vi "Dashboard Main.vi"() -> ()   [LabVIEW 2019]
uses:
  <vilib>/Utility/miscctls.llb/LVRowAndColumnTypeDef.ctl
  <vilib>/event_ctls.llb/eventvkey.ctl
  <vilib>/Rock Robotics/Network Tables/NT Read Numeric Array.vi
  <vilib>/Rock Robotics/Network Tables/NT Read Boolean.vi
  <vilib>/Rock Robotics/Network Tables/NT Read Variant.vi
  <vilib>/Rock Robotics/WPI/Dashboard/WPI_DashboardLogging Global.vi
panel:
  in  "Camera Settings Right":T1={"Frame Rate"=30, "Compression"=30, "Size"=1, "DB Camera Config"=FALSE} {"Frame Rate" scale=1.0..30.0; "Compression" scale=100.0..-1.0; "Size" items=["640x480", "320x240", "160x120"]}
  in  "Camera Name Right":string(combo)="No Camera Selection"
  out "Camera Perf":string
  in  "Camera Settings":T1={"Frame Rate"=30, "Compression"=30, "Size"=1, "DB Camera Config"=FALSE} {"Frame Rate" scale=1.0..30.0; "Compression" scale=100.0..-1.0; "Size" items=["640x480", "320x240", "160x120"]}
  in  "TCP":refnum<k5>
  in  "Rec Mode":enum32{"Stop", "Record", "Playback"}(radio)
  out "Robot IP":string
  out "Image Message":string="Timeout in Camera Communications"
  in  "Dashboard Tab":T2(tab)
  in  "Select Auto":string(combo)="Select Autonomous ..."
  out "NT Connection":bool
  out "MotorChart R":cluster{"Numeric":dbl, "Numeric":dbl}(graph)
  out "MotorChart L":cluster{"Numeric":dbl, "Numeric":dbl}(graph)
  out "MotorSliders R":cluster{"MotorSlide1":dbl, "MotorSlide2":dbl} {"MotorSlide2" scale=-1.0..1.0 scale format="%#_2e"; "MotorSlide1" scale=-1.0..1.0 scale format="%#_2e"}
  out "MotorSliders L":cluster{"MotorSlide1":dbl, "MotorSlide2":dbl} {"MotorSlide2" scale=-1.0..1.0 scale format="%#_2e"; "MotorSlide1" scale=-1.0..1.0 scale format="%#_2e"}
  out "Gyro":dbl(knob) scale=0.0..360.0
  out "JS1 Z":dbl(slide) scale=-1.0..1.0 scale format="%#_2e"
  out "JS1 Graph":cluster{"X":dbl, "Y":dbl}[](graph)
  out "JS1 Buttons":T3
  out "JS2 Z":dbl(slide) scale=-1.0..1.0 scale format="%#_2e"
  out "JS2 Graph":cluster{"X":dbl, "Y":dbl}[](graph)
  out "JS2 Buttons":T3
  out "Mode":T4(ring)=enum."Auto Disabled"
  out "Right Camera Perf":cluster{"Bandwidth (Mbps)":dbl, "FPS":dbl}
  out "Camera Image Right":T5(plugin-control)
  in  "DB/String 9":string
  in  "DB/String 8":string
  in  "DB/String 7":string
  in  "DB/String 6":string
  in  "DB/String 5":string
  in  "DB/String 4":string
  in  "DB/String 3":string
  in  "DB/String 2":string
  in  "DB/String 1":string
  in  "DB/String 0":string
  in  "DB/Slider 0":dbl(slide) scale=0.0..5.0
  in  "DB/Slider 1":dbl(slide) scale=0.0..5.0
  in  "DB/Slider 2":dbl(slide) scale=0.0..5.0
  in  "DB/Slider 3":dbl(slide) scale=0.0..5.0
  out "DB/LED 3":bool
  out "DB/LED 2":bool
  out "DB/LED 1":bool
  out "DB/LED 0":bool
  in  "DB/Button 3":bool
  in  "DB/Button 2":bool
  in  "DB/Button 1":bool
  in  "DB/Button 0":bool caption="New Name"
  out "Unjam?":bool
  out "Turret State":T6
  out "Safe for Trench?":bool
  out "Feeder State":T7
  in  "Test Slider":dbl(slide) scale=0.0..100.0 scale format="%#_3g"
  in  "On/Off":bool caption="Solenoid"
  in  "Test Name":u16(ring) items=["Select the test to run..."]
  in  "Test Tree":string(tree)
  in  "Motor":cluster{"Value":dbl, "Enable":bool} {"Value" scale=-1.0..1.0 scale format="%#_3g"}
  out "Progress":T8 {"Test Progress" scale=0.0..100.0}
  in  "Rev/Fwd":cluster{"Forward":bool, "Reverse":bool}
  in  "Test Ring":u16(ring) items=["Monochrome", "Color"]
  out "Cmd Status":string
  in  "Execute Command":bool
  in  "Command Params":string[][](table)
  in  "Command Selection":i32(listbox)
  in  "CheckList":i32(listbox)
  out "Tree":string(tree)
  out "Camera Image":T5(plugin-control)
  out "Background":bool
  in  "Camera Name":string(combo)="No Camera Selection"
  # "HW"
  # "HW"
  # "Joysticks"
  # "Drive Motors"
  # "Front"
  # "Right"
  # "Left"
  # "Back"
  # "Safe for Trench?"
  # "Feeder State"
  # "Turret State"
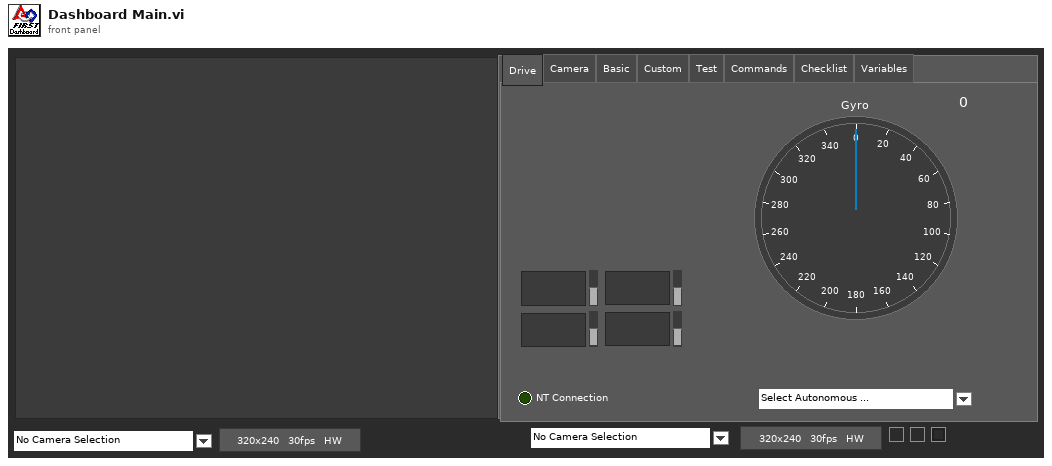
[diagram p1: front panel]
types:
  T1 = cluster{"Frame Rate":i32, "Compression":i32, "Size":u16, "DB Camera Config":bool}
  T2 = enum32{"Drive", "Camera", "Basic", "Custom", "Test", "Commands", "Checklist", "Variables"}
  T3 = cluster{bool, bool, bool, bool, bool, bool, bool, bool, bool, bool, bool, bool}
  T4 = enum8{"Tele-Op Disabled", "Tele-Op Enabled", "Auto Disabled", "Auto Enabled", "Test Disabled", "Test Enabled", "Disconnected", "No Code", "E-Stop"}
  T5 = typedef "IMAQ Image.ctl" = refnum<image>
  T6 = cluster{"Shooter Up To Speed?":bool, "Aligned With Target?":bool, "Hood at Angle?":bool, "Shooting?":bool, "Hood Angle":dbl, "Turret Angle":dbl, "Shooter Velocity":dbl}
  T7 = cluster{"Feeder Up to Speed? ":bool, "Index Clear?":bool}
  T8 = cluster{"Test Progress":u8, "Test Progress Text":string}
  T9 = cluster{"Save Path":path, "Interval (s)":dbl, "Keep":i32}
  T10 = typedef "Image Type" = u32
  T11 = cluster{"IDs":cluster{"RPC field ID":u16, "Unique ID":u16}, "String":string}
  T12 = cluster{"Error Strings":string, "Disable Counts":cluster{u16, u16}, "Rail Faults":cluster{u16, u16, u16}, "Robot IP":string, "DB Mode":u8, "Event Info":cluster{"Name":string, "Type":u8, "Number":u16, "Replay":u8}}
  T13 = cluster{"Storage":cluster{"Disk Free":u64, "RAM Block":u32, "RAM free":u32}, "CPU Utilization":cluster{"CPU % ISR":sgl, "CPU % Time Crit":sgl, "CPU % Timed Str":sgl, "CPU % High":sgl, "CPU % Above":sgl, "CPU % Normal":sgl, "CPU % Low":sgl}, "CAN":cluster{"% Bus Utilization":sgl, "Bus Off Cnt":u32, "TX_FIFO Full Cnt":u32, "Receive Error Cnt":u8, "Transmit Error Cnt":u8}, "HID":cluster{"HID Outputs":u32, "Rumble Low":u16, "Rumble High":u16}[]}
  T14 = cluster{"Status bits":cluster{"Test Mode":bool, "Autonomous":bool, "Enabled":bool, "Code Start":bool, "Brownout":bool, "Reserved 2":bool, "Reserved 3":bool, "E-Stop":bool}, "Code Trace":cluster{"Disabled":bool, "TeleOp":bool, "Auto":bool, "Test":bool}, "Controller Type":enum16{"unknown", "cRIO", "roboRio"}, "Code?":enum16{"unknown", "noCode", "code"}, "Battery V":dbl}
  T15 = cluster{"Control Bits":cluster{"TestMode":bool, "Autonomous":bool, "Enabled":bool, "FMS Present":bool, bool, bool, bool, "E-Stop":bool}, "Team Station ":u8, "Countdown":sgl, "Joystick Values":cluster{"Axes":dbl[], "Buttons":bool[], "POVs":i16[]}[]}
  T16 = cluster{"Axes":dbl[], "Buttons":bool[], "POVs":i16[]}[]
  T17 = cluster{"Axes":dbl[], "Buttons":bool[], "POVs":i16[]}
  T18 = cluster{"Buttons[0]":bool, "Buttons[1]":bool, "Buttons[2]":bool, "Buttons[3]":bool, "Buttons[4]":bool, "Buttons[5]":bool, "Buttons[6]":bool, "Buttons[7]":bool, "Buttons[8]":bool, "Buttons[9]":bool, "Buttons[10]":bool, "Buttons[11]":bool}
  T19 = cluster{"Camera Image":refnum<vi>, "Dashboard Tab":refnum<vi>, "Background":refnum<vi>, "Rec Mode":refnum<vi>, "Test Slider":refnum<vi>, "On/Off ":refnum<vi>, "Test Ring":refnum<vi>, "Rev/Fwd":refnum<vi>, "Test Name":refnum<vi>, "Motor":refnum<vi>, "Progress":refnum<vi>, "CheckList":refnum<vi>, "Tree":refnum<vi>, "Test Tree":refnum<vi>, "Command Params":refnum<vi>, "Command Selection":refnum<vi>, "Execute Command":refnum<vi>, "Cmd Status":refnum<vi>, "Camera Settings":refnum<vi>, "Camera Name":refnum<vi>, "Camera Perf":refnum<vi>, "Camera Settings Right":refnum<vi>, "Camera Name Right":refnum<vi>, "Camera Image Right":refnum<vi>}
  T20 = cluster{"Global Rectangle":i32[], "Contours":cluster{"Contour Type":u32, "ROI Type":u32, "Points":i32[]}[]}
  T21 = cluster{"Camera Name":string, string, "Saved DB Images Info":cluster{"Save Path":path, "Interval (s)":dbl, "Keep":i32}}
  T22 = cluster{"Camera Name Right":string, string, "Saved DB Images Info":cluster{"Save Path":path, "Interval (s)":dbl, "Keep":i32}}
  T23 = cluster{"Operation":enum16{"Update", "Clear"}, "Color Box":u32}[]
  T24 = typedef "eventvkey.ctl" = enum16{"ASCII", "Enter", "Return", "Shift", "Ctrl", "Alt", "Cmd", "Opt", "Caps", "NumLock", "Clear", "Break", "Up", "Down", "Left", "Right", "Insert", "Delete", "Home", "End", "PageUp", "PageDown", "Escape", "Help", "Pause", "ScrollLock", "F1", "F2", "F3", "F4", "F5", "F6", "F7", "F8", "F9", "F10", "F11", "F12", "F13", "F14", "F15", "F16", "F17", "F18", "F19", "F20", "F21", "F22", "F23", "F24", "Play", "VolumeUp", "VolumeDown", "Mute", "Two Byte Char"}
  T25 = cluster{"Image Size":bool, "Image Type":bool, "Pixel Value":bool, "ROI Information":bool, "Zoom Factor":bool}
  T26 = cluster{"Operation":enum16{"Update", "Clear"}, "Color Box":u32}
  T27 = typedef "LVRowAndColumnTypeDef.ctl" = cluster{"Row":i32, "Column":i32}
  T28 = cluster{"Shift":bool, "Ctrl":bool, "Alt":bool, "Cmd":bool, "Opt":bool}
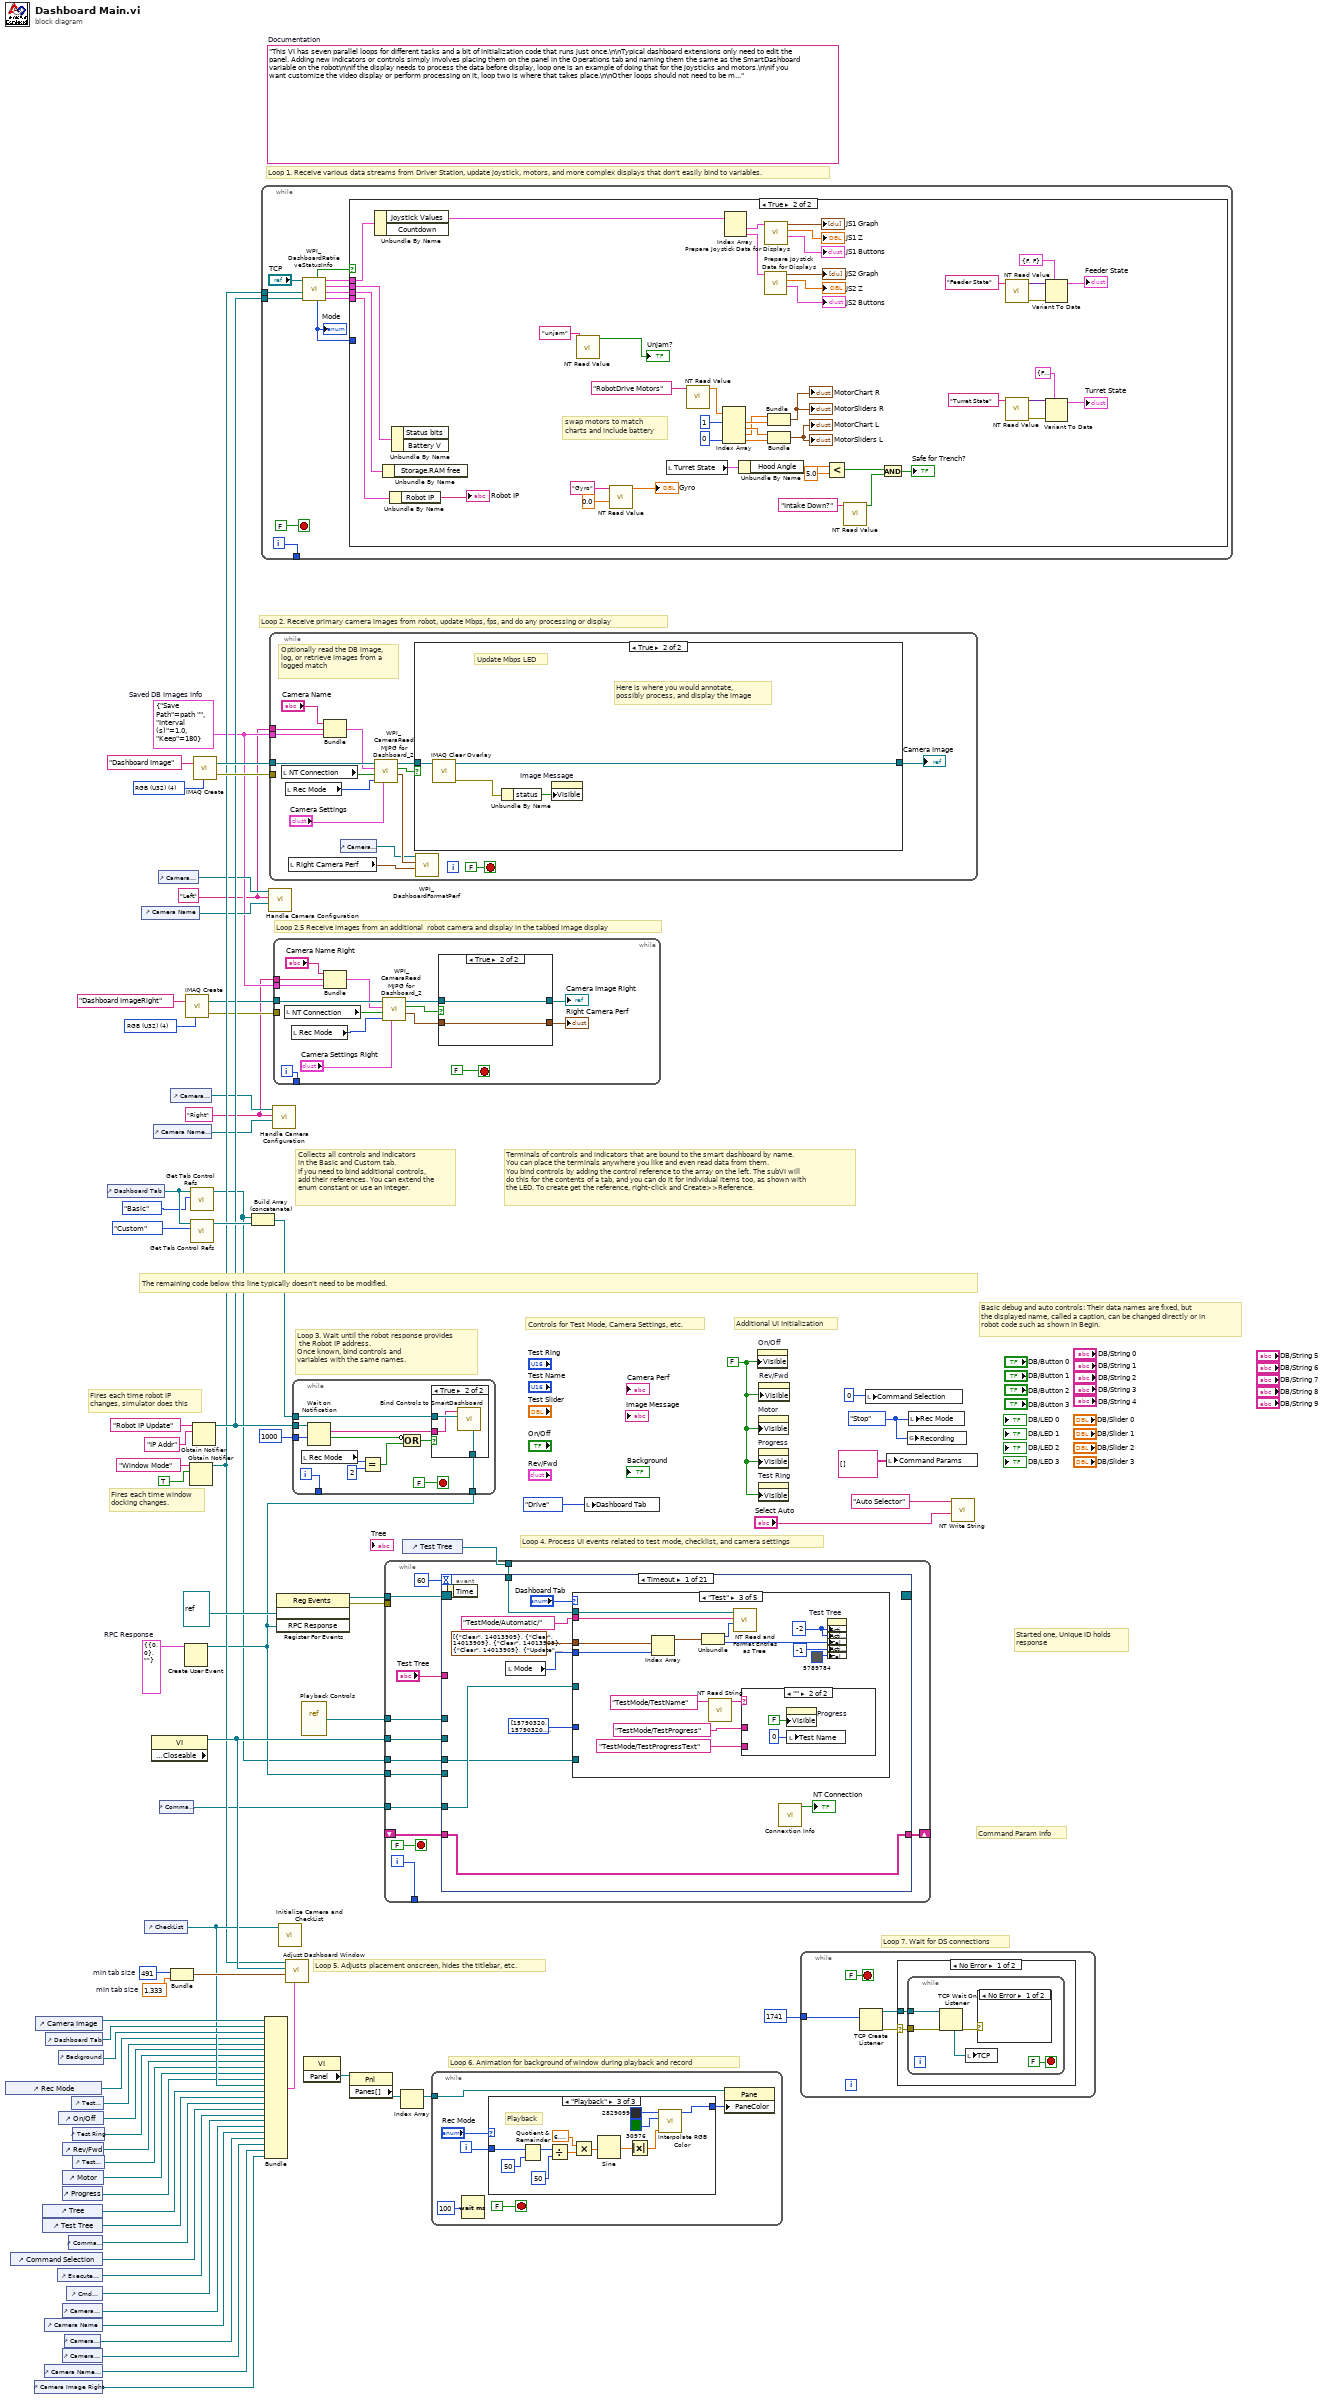
[diagram p0: block diagram]
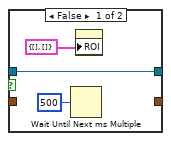
[diagram p2: hidden frame]
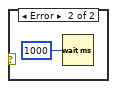
[diagram p3: hidden frame]
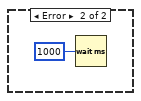
[diagram p4: hidden frame]
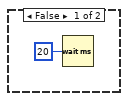
[diagram p5: hidden frame]
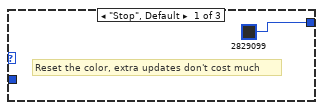
[diagram p6: hidden frame]
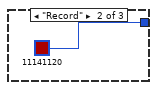
[diagram p7: hidden frame]
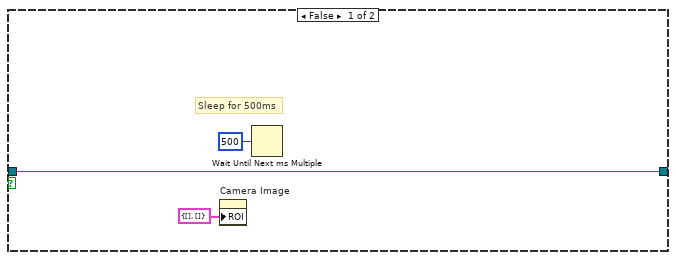
[diagram p9: hidden frame]
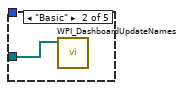
[diagram p11: hidden frame]
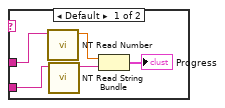
[diagram p12: hidden frame]
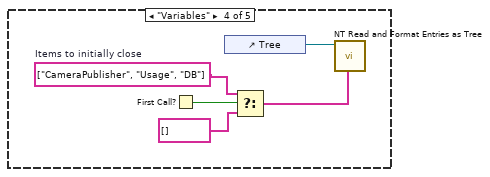
[diagram p13: hidden frame]
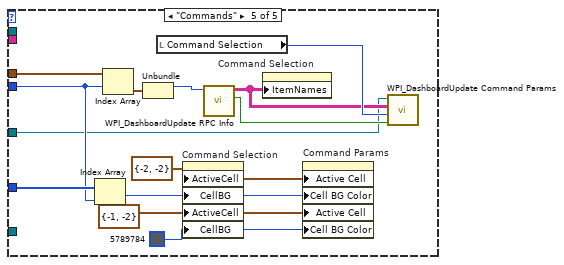
[diagram p14: hidden frame]
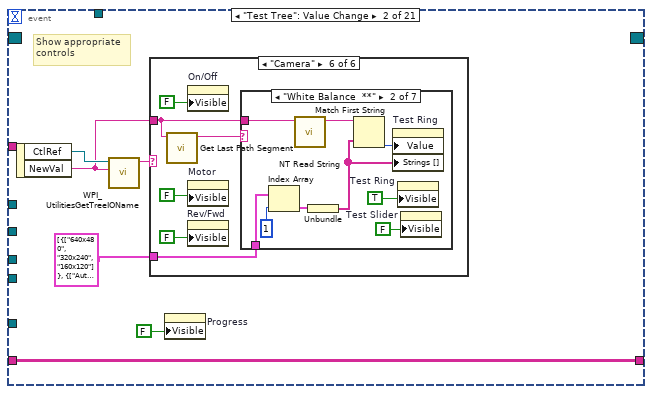
[diagram p15: hidden frame]
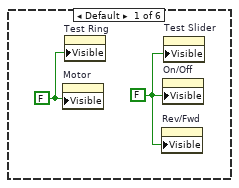
[diagram p16: hidden frame]
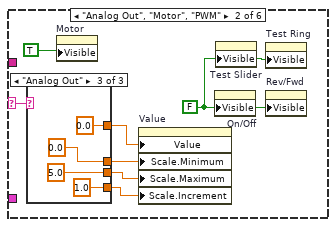
[diagram p17: hidden frame]
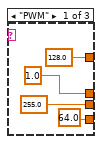
[diagram p18: hidden frame]
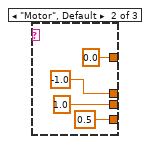
[diagram p19: hidden frame]
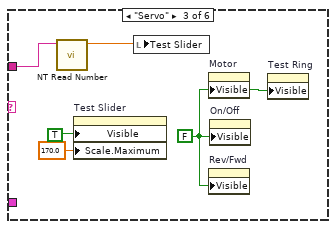
[diagram p20: hidden frame]
diagram:
  w3 = T9 {"Save Path"=path "", "Interval (s)"=1.0, "Keep"=180}  # Saved DB Images Info
  w2 = "Right"
  w1 = "Left"
  w13 = T10 4 items=["Grayscale (U8)", "Grayscale (I16)", "Grayscale (SGL)", "Complex (CSG)", "RGB (U32)", "HSL (U32)", "RGB (U64)"] ("Image Type")
  w29 = T11 {"IDs"={"RPC field ID"=0, "Unique ID"=0}, "String"=""}  # RPC Response
  w52 = 491  # min tab size
  w51 = 1.333  # min tab size
  w59 = enum32{"Stop", "Record", "Playback"}."Stop" ("Rec Mode")
  w36 = FALSE ("Visible")
  (unwired) "This VI has seven parallel loops for different tasks and a bit of initialization code that runs just once.\n\nTypical dashboard extensions only need to edit the panel. Adding new indicators or controls simply involves placing them on the panel in the Operations tab and naming them the same as the SmartDashboard variable on the robot\n\nIf the display needs to process the data before display, loop one is an example of doing that for the joysticks and motors.\n\nIf you want customize the video display or perform processing on it, loop two is where that takes place.\n\nOther loops should not need to be modified. They are pretty standard, and document the task they perform."  # Documentation
  w76 = T10 4 items=["Grayscale (U8)", "Grayscale (I16)", "Grayscale (SGL)", "Complex (CSG)", "RGB (U32)", "HSL (U32)", "RGB (U64)"] ("Image Type")
  # "Loop 2.5 Receive images from an additional  robot camera and display in the tabbed image display"
  # "Command Param Info"
  # "Started one, Unique ID holds\nresponse"
  # "Loop 7. Wait for DS connections"
  # "Basic debug and auto controls: Their data names are fixed, but\nthe displayed name, called a caption, can be changed directly or in\nrobot code such as shown in Begin."
  # "Controls for Test Mode, Camera Settings, etc."
  # "Additional UI Initialization"
  # "Loop 6. Animation for background of window during playback and record"
  # "Fires each time robot IP\nchanges, simulator does this"
  # "Fires each time window\ndocking changes."
  # "Collects all controls and indicators\nin the Basic and Custom tab.\nIf you need to bind additional controls,\nadd their references. You can extend the\nenum constant or use an integer."
  # "The remaining code below this line typically doesn't need to be modified."
  # "Loop 4. Process UI events related to test mode, checklist, and camera settings"
  # "Terminals of controls and indicators that are bound to the smart dashboard by name.\nYou can place the terminals anywhere you like and even read data from them.\nYou bind controls by adding the control reference to the array on the left. The subVI will\ndo this for the contents of a tab, and you can do it for individual items too, as shown with\nthe LED. To create get the reference, right-click and Create>>Reference."
  # "Loop 3. Wait until the robot response provides\n the Robot IP address.\nOnce known, bind controls and\nvariables with the same names."
  # "Loop 5. Adjusts placement onscreen, hides the titlebar, etc."
  # "Loop 1. Receive various data streams from Driver Station, update joystick, motors, and more complex displays that don't easily bind to variables."
  # "Loop 2. Receive primary camera images from robot, update Mbps, fps, and do any processing or display"
  n1 = control-ref of="Rec Mode"() -> (w42:refnum<vi>)
  n2 = control-ref of="Command Selection"() -> (w28:refnum<vi>)
  n3 = control-ref of="Camera Image Right"() -> (w6:refnum<vi>)
  n4 = control-ref of="Camera Image"() -> (w54:refnum<vi>)
  n5 = control-ref of="Tree"() -> (w46:refnum<vi>)
  n6 = control-ref of="Test Tree"() -> (w45:refnum<vi>)
  n7 = control-ref of="Camera Name"() -> (w19:refnum<vi>)
  n8 = control-ref of="Camera Name Right"() -> (w7:refnum<vi>)
  n9 = control-ref of="Dashboard Tab"() -> (w53:refnum<vi>)
  n10 = control-ref of="Execute Command"() -> (w30:refnum<vi>)
  n11 = control-ref of="Background"() -> (w49:refnum<vi>)
  n12 = control-ref of="On/Off"() -> (w40:refnum<vi>)
  n13 = control-ref of="Progress"() -> (w37:refnum<vi>)
  n14 = control-ref of="Camera Settings"() -> (w20:refnum<vi>)
  n15 = control-ref of="Camera Settings Right"() -> (w8:refnum<vi>)
  n16 = control-ref of="Rev/Fwd"() -> (w38:refnum<vi>)
  n17 = control-ref of="Motor"() -> (w43:refnum<vi>)
  n18 = control-ref of="Camera Perf"() -> (w18:refnum<vi>)
  n19 = control-ref of="Cmd Status"() -> (w24:refnum<vi>)
  n20 = control-ref of="Command Params"() -> (w31:refnum<vi>)
  n21 = control-ref of="Test Slider"() -> (w41:refnum<vi>)
  n22 = control-ref of="Test Ring"() -> (w39:refnum<vi>)
  n23 = control-ref of="Test Name"() -> (w44:refnum<vi>)
  n24 = control-ref of="Dashboard Tab"() -> (w57:refnum<vi>)
  n25 = control-ref of="Camera Name"() -> (w21:refnum<vi>)
  n26 = control-ref of="CheckList"() -> (w47:refnum<vi>)
  n27 = property class="VI" props=["Front Panel.Closeable"]() -> (reference out=w58:refnum<vi>)  [unwired: 2 in, 2 out]
  n28 = control-ref of="Camera Name Right"() -> (w9:refnum<vi>)
  n29 = control-ref of="Camera Settings"() -> (w22:refnum<vi>)
  n30 = control-ref of="Command Params"() -> (w23:refnum<vi>)
  n31 = control-ref of="Camera Settings Right"() -> (w10:refnum<vi>)
  n32 = Bundle("min tab size"=w52, "min tab size"=w51) -> (w50:cluster{"min tab size":i32, "min tab size":dbl})  [unwired: 1 in]
  n33 = Create User Event(user event datatype=w29) -> (user event=w25:refnum<user-event>)  [unwired: 1 in, 1 out]
  n34 = call "IMAQ Create"("Image Name"="Dashboard ImageRight", "Image Type"=w13) -> ("New Image"=w12:T5, "error out"=w11:errorcluster)  [unwired: 2 in, 1 out]
  n35 = Obtain Notifier(name (unnamed)="Window Mode", notification data type=TRUE) -> (notifier out=w34:refnum<notifier>)  [unwired: 2 in, 2 out]
  n36 = call <vilib>:"Get Tab Control Refs.vi"("Page Index"=T2."Basic" ("Dashboard Tab"), "TabControl in"=w57) -> ("ControlsOnPage"=w17:refnum<vi>[])  [unwired: 9 in]
  n37 = call <vilib>:"Get Tab Control Refs.vi"("Page Index"=T2."Custom" ("Dashboard Tab"), "TabControl in"=w57) -> ("ControlsOnPage"=w56:refnum<vi>[])  [unwired: 9 in]
  n38 = Obtain Notifier(name (unnamed)="Robot IP Update", notification data type="IP Addr" ("name (unnamed)")) -> (notifier out=w35:refnum<notifier>)  [unwired: 2 in, 2 out]
  n39 = call "IMAQ Create"("Image Name"="Dashboard Image", "Image Type"=w76) -> ("New Image"=w74:T5, "error out"=w73:errorcluster)  [unwired: 2 in, 1 out]
  n40 = Build Array (concatenate)(w17, w56) -> (w55:refnum<vi>[])
  n41 = while {
    tunnel: [w86] -> _
    tunnel: w35 -> [w80]
    tunnel: w34 -> [w77]
    i -> [w86]
    stop <- FALSE stop-if-true
    n42 = call <vilib>:"WPI_DashboardRetrieveStatusInfo.vi"("Binding Refnum"=w80, "Window Mode Notifier"=w77, "TCP Cnx"="TCP") -> ("Power and Errors"=w81:T12, "Robot Metrics"=w84:T13, "Status Info"=w85:T14, "Control Info"=w82:T15, "Robot Mode"=w79:T4, "Process?"=w83:bool)  [unwired: 3 in]
    "Mode" <- w79
    n43 = case shown="True" w83 {
      tunnel: w85 -> [_ w134]
      tunnel: w84 -> [_ w133]
      tunnel: w82 -> [_ w132]
      tunnel: w81 -> [_ w131]
      tunnel: w79 -> [_ _]
      frame False {
        n44 = Wait (ms)(milliseconds to wait=u32 20) -> ()  [unwired: 1 out]
      }
      frame True {
        # "swap motors to match\ncharts and include battery"
        n45 = Unbundle By Name(w132) -> ("Joystick Values"=w122:T16)  [unwired: 1 out]
        n46 = Unbundle By Name(w133) -> ()  [unwired: 1 out]
        n47 = Unbundle By Name(w131) -> ("Robot IP"=→"Robot IP":string)
        n48 = Unbundle By Name(w134) -> ()  [unwired: 2 out]
        n49 = call-poly <vilib>:"NT Read Value.vi"("Name"="unjam") -> ("Boolean"=→"Unjam?":bool)  [unwired: 9 in, 1 out]
        n50 = call-poly <vilib>:"NT Read Value.vi"("Default Value"=0.0, "Name"="Gyro") -> ("Numeric"=→"Gyro":dbl)  [unwired: 8 in, 1 out]
        n51 = local read "Turret State"() -> (w95:T6)
        n52 = call-poly <vilib>:"NT Read Value.vi"("Name"="RobotDrive Motors") -> ("Numeric Array"=w112:dbl[])  [unwired: 9 in, 1 out]
        n53 = Index Array(array=w112, index #1=1, index #4=0) -> (element #1=w126:dbl, element #2=w127:dbl, element #3=w125:dbl, element #4=w130:dbl)  [unwired: 2 in]
        n54 = Index Array(array=w122) -> (element #1=w121:T17, element #2=w117:T17)  [unwired: 2 in]
        n55 = Unbundle By Name(w95) -> ("Hood Angle"=w93:dbl)
        n56 = call "Prepare Joystick Data for Displays.vi"("Joystick Values"=w117) -> ("Buttons"=→"JS2 Buttons":T18, "Z Axis"=→"JS2 Z":dbl, "Cartesian Data"=→"JS2 Graph":cluster{"X axis":dbl, "X axis":dbl}[])  [unwired: 8 in]
        n57 = call "Prepare Joystick Data for Displays.vi"("Joystick Values"=w121) -> ("Buttons"=→"JS1 Buttons":T18, "Z Axis"=→"JS1 Z":dbl, "Cartesian Data"=→"JS1 Graph":cluster{"X axis":dbl, "X axis":dbl}[])  [unwired: 8 in]
        n58 = Bundle("Numeric"=w125, "Numeric"=w126) -> (→"MotorChart R" →"MotorSliders R":cluster{"Numeric":dbl, "Numeric":dbl})  [unwired: 1 in]
        n59 = Bundle("Numeric"=w127, "Numeric"=w130) -> (→"MotorChart L" →"MotorSliders L":cluster{"Numeric":dbl, "Numeric":dbl})  [unwired: 1 in]
        n60 = Less?(x=w93, y=5.0) -> (x < y?=w91:bool)
        n61 = call-poly <vilib>:"NT Read Value.vi"("Name"="Intake Down?") -> ("Boolean"=w106:bool)  [unwired: 9 in, 1 out]
        n62 = And(x=w91, y=w106) -> (x .and. y?=→"Safe for Trench?":bool)
        n63 = call-poly <vilib>:"NT Read Value.vi"("Name"="Feeder State") -> ("error out"=w98:errorcluster, "Variant"=w104:variant)  [unwired: 9 in]
        n64 = call-poly <vilib>:"NT Read Value.vi"("Name"="Turret State") -> ("error out"=w99:errorcluster, "Variant"=w100:variant)  [unwired: 9 in]
        n65 = Variant To Data(error in=w98, type=T7 {"Feeder Up to Speed? "=FALSE, "Index Clear?"=FALSE} ("Feeder State"), Variant=w104) -> (data=→"Feeder State":T7)  [unwired: 1 out]
        n66 = Variant To Data(error in=w99, type=T6 {"Shooter Up To Speed?"=FALSE, "Aligned With Target?"=FALSE, "Hood at Angle?"=FALSE, "Shooting?"=FALSE, "Hood Angle"=0.0, "Turret Angle"=0.0, "Shooter Velocity"=0.0} ("Turret State"), Variant=w100) -> (data=→"Turret State":T6)  [unwired: 1 out]
      }
    }
  }
  n67 = Bundle("Camera Image"=w54, "Dashboard Tab"=w53, "Background"=w49, "Rec Mode"=w42, "Test Slider"=w41, "On/Off"=w40, "Test Ring"=w39, "Rev/Fwd"=w38, "Test Name"=w44, "Motor"=w43, "Progress"=w37, "CheckList"=w47, "Tree"=w46, "Test Tree"=w45, "Command Params"=w31, "Command Selection"=w28, "Execute Command"=w30, "Cmd Status"=w24, "Camera Settings"=w20, "Camera Name"=w19, "Camera Perf"=w18, "Camera Settings Right"=w8, "Camera Name Right"=w7, "Camera Image Right"=w6) -> (w48:T19)  [unwired: 1 in]
  n68 = call "Handle Camera Configuration.vi"("CameraNameRef"=w21, "Display Name"=w1, "ClusterRef"=w22) -> ()  [unwired: 9 in]
  n69 = while {
    tunnel: w74 -> [w148]
    tunnel: w73 -> [_]
    tunnel: w3 -> [w141]
    tunnel: w1 -> [w138]
    stop <- FALSE stop-if-true
    # "Optionally read the DB image,\nlog, or retrieve images from a\nlogged match"
    n70 = local read "NT Connection"() -> (w142:bool)
    n71 = local read "Rec Mode"() -> (w145:enum32{"Stop", "Record", "Playback"})
    n72 = local read "Right Camera Perf"() -> (w136:cluster{"Bandwidth (Mbps)":dbl, "FPS":dbl})
    n73 = Bundle("Camera Name"="Camera Name", w138, "Saved DB Images Info"=w141) -> (w140:T21)  [unwired: 1 in]
    n74 = control-ref of="Camera Perf"() -> (w135:refnum<vi>)
    n75 = call <vilib>:"WPI_CameraRead MJPG for Dashboard_2.vi"("Camera Settings"="Camera Settings", "Rec Mode"=w145, "NT Connection"=w142, "Capture Info"=w140, "Image in"=w148) -> ("perf info"=w137:cluster{"Bandwidth (Mbps)":dbl, "fps":dbl}, "Active"=w146:bool, "Image\\ out"=w147:T5)  [unwired: 4 in]
    n76 = case shown="True" w146 {
      tunnel: w147 -> [w151 w154]
      tunnel: [w151 w153] -> w143
      frame False {
        # "Sleep for 500ms"
        n77 = property on="Camera Image" class="ImageControl"("ROI"=T20 {"Global Rectangle"=[], "Contours"=[]}) -> ()  [unwired: 2 in, 2 out]
        n78 = Wait Until Next ms Multiple(millisecond multiple=u32 500) -> ()  [unwired: 1 out]
      }
      frame True {
        # "Here is where you would annotate,\npossibly process, and display the image"
        # "Update Mbps LED"
        n79 = call "IMAQ Clear Overlay"("Image"=w154) -> ("error out"=w155:errorcluster, "Image Out"=w153:T5)  [unwired: 2 in, 7 out]
        n80 = Unbundle By Name(w155) -> ("status"=w156:bool)
        n81 = property on="Image Message" class="Str"("Visible"=w156) -> ()  [unwired: 2 in, 2 out]
      }
    }
    "Camera Image" <- w143
    n82 = call <vilib>:"WPI_DashboardFormatPerf.vi"("Right Camera Perf"=w136, "Performance"=w137, "String in"=w135) -> ()  [unwired: 9 in]
  }
  n83 = call "Handle Camera Configuration.vi"("CameraNameRef"=w9, "Display Name"=w2, "ClusterRef"=w10) -> ()  [unwired: 9 in]
  n84 = while {
    tunnel: w12 -> [w171]
    tunnel: w11 -> [_]
    tunnel: [w166] -> _
    tunnel: w3 -> [w162]
    tunnel: w2 -> [w159]
    i -> [w166]
    stop <- FALSE stop-if-true
    n85 = local read "NT Connection"() -> (w163:bool)
    n86 = local read "Rec Mode"() -> (w170:enum32{"Stop", "Record", "Playback"})
    n87 = Bundle("Camera Name Right"="Camera Name Right", w159, "Saved DB Images Info"=w162) -> (w161:T22)  [unwired: 1 in]
    n88 = call <vilib>:"WPI_CameraRead MJPG for Dashboard_2.vi"("Camera Settings"="Camera Settings Right", "Rec Mode"=w170, "NT Connection"=w163, "Capture Info"=w161, "Image in"=w171) -> ("perf info"=w157:cluster{"Bandwidth (Mbps)":dbl, "fps":dbl}, "Active"=w165:bool, "Image\\ out"=w168:T5)  [unwired: 4 in]
    n89 = case shown="True" w165 {
      tunnel: w168 -> [w173 w176]
      tunnel: [w173 w176] -> w164
      tunnel: [_ w175] -> w158
      tunnel: w157 -> [_ w175]
      frame False {
        n90 = Wait Until Next ms Multiple(millisecond multiple=u32 500) -> ()  [unwired: 1 out]
        n91 = property on="Camera Image Right" class="ImageControl"("ROI"=T20 {"Global Rectangle"=[], "Contours"=[]}) -> ()  [unwired: 2 in, 2 out]
      }
      frame True {
      }
    }
    "Camera Image Right" <- w164
    "Right Camera Perf" <- w158
  }
  n92 = register-events(refnum<vi> refnum, w25) -> (reference out=w63:refnum<event-registration>, error out=w62:errorcluster)  [unwired: 2 in]
  n93 = call "Initialize Camera and CheckList.vi"("ListBox in"=w47) -> ()  [unwired: 11 in]
  n94 = call "Adjust Dashboard Window.vi"("Sizing Refnums"=w48, "Size Constraints"=w50, "VI"=w58, "WIn Mode"=w34) -> ()  [unwired: 8 in]
  n95 = while {
    tunnel: w55 -> [w188]
    tunnel: w35 -> [w186]
    tunnel: [w184] -> _
    tunnel: u32 1000 ("milliseconds to wait") -> [w183]
    tunnel: w25 -> [w177]
    i -> [w184]
    stop <- FALSE stop-if-true
    n96 = local read "Rec Mode"() -> (w179:enum32{"Stop", "Record", "Playback"})
    n97 = Wait on Notification(notifier=w186, timeout in ms (-1)=w183) -> (notification=w185:string, timed out?=w181:bool)  [unwired: 2 in, 2 out]
    n98 = Equal?(x=w179, y=u16 2 ("Rec Mode")) -> (x = y?=w180:bool)
    n99 = Compound Arithmetic op=OR(invert w181, w180) -> (w182:bool)
    n100 = case shown="True" w182 {
      tunnel: w188 -> [_ w191]
      tunnel: w185 -> [_ w190]
      tunnel: w177 -> [_ w189]
      frame False {
      }
      frame True {
        n101 = call <vilib>:"Bind Controls to SmartDashboard.vi"("RPC ref"=w189, "Bound Control Refs"=w191, "Server IP Address"=w190) -> ()  [unwired: 9 in]
      }
    }
  }
  n102 = vi-ref "Playback Controls.vi"() -> (w64:refnum<vi>)
  n103 = property class="VI"() -> ("Panel"=w66:refnum<vi>)  [unwired: 2 in, 2 out]
  n104 = property class="Pnl"(reference=w66) -> ("Panes[]"=w67:refnum<vi>[])  [unwired: 1 in, 2 out]
  n105 = Index Array(array=w67) -> (element=w65:refnum<vi>)  [unwired: 1 in]
  n106 = control-ref of="Test Tree"() -> (w68:refnum<vi>)
  n107 = while {
    tunnel: [w201] -> _
    tunnel: w68 -> [w200]
    tunnel: w64 -> [w199]
    tunnel: w63 -> [w198]
    tunnel: w62 -> [_]
    tunnel: w58 -> [w197]
    tunnel: w25 -> [w196]
    tunnel: w23 -> [w195]
    shift-right: [w194] -> _
    shift-left: _ -> [w193]
    tunnel: w17 -> [w192]
    i -> [w201]
    stop <- FALSE stop-if-true
    n108 = event shown="[0] Timeout" {
      selector: w198 -> [_ _ _ _ _ _ _ _ _ _ _ _ _ _ _ _ _ _ _ _ _]
      dyn-events: [_ _ _ _ _ _ _ _ _ _ _ _ _ _ _ _ w461 _ _ _ _] -> _
      timeout: u32 60 ("milliseconds to wait") -> [_ _ _ _ _ _ _ _ _ _ _ _ _ _ _ _ _ _ _ _ _]
      tunnel: w200 -> [w213 _ _ _ _ _ _ _ _ _ _ _ _ _ _ _ _ _ _ _ _]
      tunnel: "Test Tree" -> [_ _ _ _ _ _ _ _ _ _ _ w428 w436 w438 w442 w450 _ _ _ _ _]
      tunnel: w199 -> [_ _ _ _ _ _ _ _ _ _ _ _ _ _ _ _ w463 _ w481 _ _]
      tunnel: w197 -> [_ _ _ _ _ _ _ _ _ _ _ _ _ _ _ _ w459 _ _ _ _]
      tunnel: w196 -> [_ _ _ _ _ _ _ _ _ _ _ _ _ _ _ _ w457 _ _ _ _]
      tunnel: w195 -> [w208 _ _ _ _ _ w379 _ _ _ _ _ _ _ _ _ _ _ _ _ _]
      tunnel: [w207 w256 w358 w363 w372 w376 w377 w386 w396 w403 w415 w427 w434 w437 w441 w449 w456 w476 w478 w482 w495] -> w194
      tunnel: w193 -> [w207 w256 w358 w363 w372 w376 w377 _ _ w403 w415 w427 w434 w437 w441 w449 w456 w476 w478 w482 w495]
      tunnel: w192 -> [w205 _ _ _ _ _ _ _ _ _ _ _ _ _ _ _ _ _ _ _ _]
      event Timeout {
        n109 = event-data() -> ()  [unwired: 1 in, 1 out]
        n110 = local read "Mode"() -> (w210:T4)
        n111 = case shown="\"Test\"" "Dashboard Tab" {
          tunnel: w213 -> [_ _ w229 _ _]
          tunnel: "TestMode/Automatic/" ("Name Pattern") -> [_ _ w228 _ _]
          tunnel: T23 [{"Operation"=enum."Clear", "Color Box"=14013909}, {"Operation"=enum."Clear", "Color Box"=14013909}, {"Operation"=enum."Clear", "Color Box"=14013909}, {"Operation"=enum."Clear", "Color Box"=14013909}, {"Operation"=enum."Update", "Color Box"=14013909}, {"Operation"=enum."Update", "Color Box"=16777215}, {"Operation"=enum."Clear", "Color Box"=14013909}, {"Operation"=enum."Clear", "Color Box"=14013909}, {"Operation"=enum."Clear", "Color Box"=14013909}] -> [_ _ w221 _ w249]
          tunnel: w210 -> [_ _ w220 _ w248]
          tunnel: u32[] [15790320, 15790320, 15790320, 15790320, 16777215, 16777215, 15790320, 15790320, 15790320] -> [_ _ _ _ w254]
          tunnel: w208 -> [_ _ _ _ w242]
          tunnel: w205 -> [_ w215 _ _ _]
          frame "Custom", Default {
          }
          frame "Basic" {
            n112 = call <vilib>:"WPI_DashboardUpdateNames.vi"("Controls on Tab"=w215) -> ()  [unwired: 11 in]
          }
          frame "Test" {
            w227 = -2 ("Active Item:Row Number")
            n113 = Index Array(array=w221, index=w220) -> (element=w222:T26)
            n114 = Unbundle(w222) -> ("Operation"=w223:enum16{"Update", "Clear"}, "Color Box"=w224:u32)
            n115 = call <vilib>:"NT Read String.vi"("Name"="TestMode/TestName") -> ("String"=w218:string)  [unwired: 9 in, 1 out]
            n116 = call <vilib>:"NT Read and Format Entries as Tree.vi"("Operation"=w223, "Name Pattern"=w228, "Tree Refnum"=w229) -> ()  [unwired: 7 in, 2 out]
            n117 = case shown="\"\"" w218 {
              tunnel: "TestMode/TestProgress" ("Name") -> [w231 _]
              tunnel: "TestMode/TestProgressText" ("Name") -> [w230 _]
              frame Default {
                n118 = call <vilib>:"NT Read Number.vi"("Name"=w231) -> ("Numeric"=w232:dbl)  [unwired: 9 in, 1 out]
                n119 = call <vilib>:"NT Read String.vi"("Name"=w230) -> ("String"=w233:string)  [unwired: 9 in, 1 out]
                n120 = Bundle("Numeric"=w232, "String"=w233) -> (→"Progress":cluster{"Numeric":dbl, "String":string})  [unwired: 1 in]
              }
              frame "" {
                n121 = property on="Progress" class="Clust (strict)"("Visible"=FALSE) -> ()  [unwired: 2 in, 2 out]
                n122 = local write "Test Name"(u16 0) -> ()
              }
            }
            n123 = property on="Test Tree" class="Tree (strict)"("Active Item Row Number"=w227, "ActiveColNum"=w227, "CellBG"=w224, "Active Item Row Number"=-1 ("Active Item:Row Number"), "CellBG"=u32 5789784 ("Color Box")) -> ()  [unwired: 2 in, 2 out]
          }
          frame "Variables" {
            w239 = string[] ["CameraPublisher", "Usage", "DB"]  # Items to initially close
            n124 = First Call?() -> (First Call?: T/F=w240:bool)
            n125 = control-ref of="Tree"() -> (w241:refnum<vi>)
            n126 = Select(t=w239, s=w240, f=string[] []) -> (s? t:f=w237:string[])
            n127 = call <vilib>:"NT Read and Format Entries as Tree.vi"("Tags to  Close"=w237, "Tree Refnum"=w241) -> ()  [unwired: 8 in, 2 out]
          }
          frame "Commands" {
            w250 = u32 5789784 ("Color Box")
            w251 = T27 {"Row"=-1, "Column"=-2} ("Active Cell:Active Cell")
            w253 = T27 {"Row"=-2, "Column"=-2} ("Active Cell:Active Cell")
            n128 = Index Array(array=w254, index=w248) -> (element=w252:u32)
            n129 = Index Array(array=w249, index=w248) -> (element=w247:T26)
            n130 = Unbundle(w247) -> ("Operation"=w246:enum16{"Update", "Clear"})  [unwired: 1 out]
            n131 = local read "Command Selection"() -> (w245:i32)
            n132 = property on="Command Selection" class="MCListbox (strict)"("ActiveCell"=w253, "CellBG"=w252, "ActiveCell"=w251, "CellBG"=w250) -> ()  [unwired: 2 in, 2 out]
            n133 = call <vilib>:"WPI_DashboardUpdate RPC Info.vi"("Operation"=w246) -> ("update"=w244:bool, "commands"=w243:string[][])  [unwired: 9 in]
            n134 = property on="Command Selection" class="MCListbox (strict)"("ItemNames"=w243) -> ()  [unwired: 2 in, 2 out]
            n135 = property on="Command Params" class="Tbl (strict)"("Active Cell"=w253, "Cell BG Color"=w252, "Active Cell"=w251, "Cell BG Color"=w250) -> ()  [unwired: 2 in, 2 out]
            n136 = call <vilib>:"WPI_DashboardUpdate Command Params.vi"("Update"=w244, "NewVal"=w245, "Commands"=w243, "Param Tbl"=w242) -> ()  [unwired: 7 in, 1 out]
          }
        }
        n137 = call <vilib>:"Connextion Info.vi"() -> ("Connected"=→"NT Connection":bool)  [unwired: 10 in, 1 out]
      }
      event "Test Tree": Value Change {
        # "Show appropriate\ncontrols"
        n138 = event-data() -> ("CtlRef"=w259:refnum<vi>, "NewVal"=w257:string)  [unwired: 1 in]
        n139 = call <vilib>:"WPI_UtilitiesGetTreeIOName.vi"("NewVal"=w257, "TreeControl in"=w259) -> ("I/O Name"=w260:string)  [unwired: 9 in]
        n140 = case shown="\"Camera\"" w260 {
          selector: w260 -> [_ w267 _ w289 w298 _]
          tunnel: w257 -> [_ _ w286 w288 _ w305]
          tunnel: cluster{string[]}[] [{["640x480", "320x240", "160x120"]}, {["Auto", "Fixed indoor", "Fixed outdoor 1", "Fixed outdoor 2", "Fixed fluorescent 1", "Fixed fluorescent 2", "Hold current"]}, {["Auto", "Flicker-free 50 Hz", "Flicker-free 60 Hz", "Hold current"]}, {["None", "Prioritize frame rate", "Prioritize image quality"]}, {["Monochrome", "Color"]}] -> [_ _ _ _ _ w304]
          frame Default {
            w262 = FALSE ("Visible")
            w261 = FALSE ("Visible")
            n141 = property on="Motor" class="Clust (strict)"("Visible"=w261) -> ()  [unwired: 2 in, 2 out]
            n142 = property on="Test Ring" class="Ring (strict)"("Visible"=w261) -> ()  [unwired: 2 in, 2 out]
            n143 = property on="Rev/Fwd" class="Clust (strict)"("Visible"=w262) -> ()  [unwired: 2 in, 2 out]
            n144 = property on="On/Off" class="Bool (strict)"("Visible"=w262) -> ()  [unwired: 2 in, 2 out]
            n145 = property on="Test Slider" class="Slide (strict)"("Visible"=w262) -> ()  [unwired: 2 in, 2 out]
          }
          frame "Analog Out", "Motor", "PWM" {
            w268 = FALSE ("Visible")
            n146 = case shown="\"Analog Out\"" w267 {
              tunnel: [1.0 ("Value") -1.0 ("Value") 0.0 ("Value")] -> w266
              tunnel: [255.0 ("Value") 1.0 ("Value") 5.0 ("Value")] -> w265
              tunnel: [128.0 ("Value") 0.0 ("Value") 0.0 ("Value")] -> w264
              tunnel: [64.0 ("Value") 0.5 ("Value") 1.0 ("Value")] -> w263
              frame "PWM" {
              }
              frame "Motor", Default {
              }
              frame "Analog Out" {
              }
            }
            n147 = property on="Motor" class="Clust (strict)"("Visible"=TRUE) -> ()  [unwired: 2 in, 2 out]
            n148 = property on="Value" class="Slide (strict)"("Value"=w264, "Scale.Minimum"=w266, "Scale.Maximum"=w265, "Scale.Increment"=w263) -> ()  [unwired: 2 in, 2 out]
            n149 = property on="On/Off" class="Bool (strict)"("Visible"=w268) -> ()  [unwired: 2 in, 2 out]
            n150 = property on="Test Slider" class="Slide (strict)"("Visible"=w268) -> ()  [unwired: 2 in, 2 out]
            n151 = property on="Test Ring" class="Ring (strict)"("Visible"=w268) -> ()  [unwired: 2 in, 2 out]
            n152 = property on="Rev/Fwd" class="Clust (strict)"("Visible"=w268) -> ()  [unwired: 2 in, 2 out]
          }
          frame "Servo" {
            w284 = FALSE ("Visible")
            n153 = call <vilib>:"NT Read Number.vi"("Name"=w286) -> ("Numeric"=w285:dbl)  [unwired: 9 in, 1 out]
            n154 = property on="Test Slider" class="Slide (strict)"("Visible"=TRUE, "Scale.Maximum"=170.0 ("Scale.Range:Maximum")) -> ()  [unwired: 2 in, 2 out]
            n155 = local write "Test Slider"(w285) -> ()
            n156 = property on="Motor" class="Clust (strict)"("Visible"=w284) -> ()  [unwired: 2 in, 2 out]
            n157 = property on="Rev/Fwd" class="Clust (strict)"("Visible"=w284) -> ()  [unwired: 2 in, 2 out]
            n158 = property on="On/Off" class="Bool (strict)"("Visible"=w284) -> ()  [unwired: 2 in, 2 out]
            n159 = property on="Test Ring" class="Ring (strict)"("Visible"=w284) -> ()  [unwired: 2 in, 2 out]
          }
          frame "Relay", "Solenoid" {
            w287 = FALSE ("Visible")
            n160 = property on="Motor" class="Clust (strict)"("Visible"=w287) -> ()  [unwired: 2 in, 2 out]
            n161 = property on="Test Slider" class="Slide (strict)"("Visible"=w287) -> ()  [unwired: 2 in, 2 out]
            n162 = Search and Replace String(input string=w288, search string="/Value  **", replace string="/Direction") -> (result string=w294:string)  [unwired: 5 in, 3 out]
            n163 = property on="Test Ring" class="Ring (strict)"("Visible"=w287) -> ()  [unwired: 2 in, 2 out]
            n164 = call <vilib>:"NT Read String.vi"("Name"=w294) -> ("String"=w292:string)  [unwired: 9 in, 1 out]
            n165 = Equal?(x="Both directions", y=w292) -> (x = y?=w290:bool)
            n166 = Not(x=w290) -> (.not. x?=w291:bool)
            n167 = property on="Rev/Fwd" class="Clust (strict)"("Visible"=w290) -> ()  [unwired: 2 in, 2 out]
            n168 = property on="On/Off" class="Bool (strict)"("Visible"=w291, "Caption.Text"=w289) -> ()  [unwired: 2 in, 2 out]
          }
          frame "Compressor", "Digital Out" {
            w297 = FALSE ("Visible")
            # "Get direction and finish"
            n169 = property on="Motor" class="Clust (strict)"("Visible"=w297) -> ()  [unwired: 2 in, 2 out]
            n170 = property on="Test Slider" class="Slide (strict)"("Visible"=w297) -> ()  [unwired: 2 in, 2 out]
            n171 = property on="Test Ring" class="Ring (strict)"("Visible"=w297) -> ()  [unwired: 2 in, 2 out]
            n172 = property on="On/Off" class="Bool (strict)"("Visible"=TRUE, "Caption.Text"=w298) -> ()  [unwired: 2 in, 2 out]
            n173 = property on="Rev/Fwd" class="Clust (strict)"("Visible"=FALSE) -> ()  [unwired: 2 in, 2 out]
          }
          frame "Camera" {
            n174 = call <vilib>:"Get Last Path Segment.vi"("String in"=w305) -> ("String out"=w306:string)  [unwired: 10 in]
            n175 = property on="On/Off" class="Bool (strict)"("Visible"=FALSE) -> ()  [unwired: 2 in, 2 out]
            n176 = property on="Motor" class="Clust (strict)"("Visible"=FALSE) -> ()  [unwired: 2 in, 2 out]
            n177 = property on="Rev/Fwd" class="Clust (strict)"("Visible"=FALSE) -> ()  [unwired: 2 in, 2 out]
            n178 = case shown="\"White Balance  **\"" w306 {
              tunnel: w305 -> [w312 w321 w330 w339 w348 _ w354]
              tunnel: w304 -> [w310 w318 w327 w336 w345 _ _]
              frame "Size  **" {
                n179 = Index Array(array=w310) -> (element=w309:cluster{string[]})  [unwired: 1 in]
                n180 = call <vilib>:"NT Read String.vi"("Name"=w312) -> ("String"=w311:string)  [unwired: 9 in, 1 out]
                n181 = Unbundle(w309) -> (w307:string[])
                n182 = Match First String(2:w307, 3:w311) -> (0:w308:i32)  [unwired: 1 out]
                n183 = property on="Test Ring" class="Ring (strict)"("Value"=w308, "Strings []"=w307) -> ()  [unwired: 2 in, 2 out]
                n184 = property on="Test Ring" class="Ring (strict)"("Visible"=TRUE) -> ()  [unwired: 2 in, 2 out]
                n185 = property on="Test Slider" class="Slide (strict)"("Visible"=FALSE) -> ()  [unwired: 2 in, 2 out]
              }
              frame "White Balance  **" {
                n186 = Index Array(array=w318, index=1) -> (element=w319:cluster{string[]})
                n187 = call <vilib>:"NT Read String.vi"("Name"=w321) -> ("String"=w320:string)  [unwired: 9 in, 1 out]
                n188 = Unbundle(w319) -> (w316:string[])
                n189 = Match First String(2:w316, 3:w320) -> (0:w315:i32)  [unwired: 1 out]
                n190 = property on="Test Ring" class="Ring (strict)"("Value"=w315, "Strings []"=w316) -> ()  [unwired: 2 in, 2 out]
                n191 = property on="Test Ring" class="Ring (strict)"("Visible"=TRUE) -> ()  [unwired: 2 in, 2 out]
                n192 = property on="Test Slider" class="Slide (strict)"("Visible"=FALSE) -> ()  [unwired: 2 in, 2 out]
              }
              frame "Exposure  **" {
                n193 = Index Array(array=w327, index=2) -> (element=w328:cluster{string[]})
                n194 = call <vilib>:"NT Read String.vi"("Name"=w330) -> ("String"=w329:string)  [unwired: 9 in, 1 out]
                n195 = Unbundle(w328) -> (w324:string[])
                n196 = Match First String(2:w324, 3:w329) -> (0:w325:i32)  [unwired: 1 out]
                n197 = property on="Test Ring" class="Ring (strict)"("Value"=w325, "Strings []"=w324) -> ()  [unwired: 2 in, 2 out]
                n198 = property on="Test Ring" class="Ring (strict)"("Visible"=TRUE) -> ()  [unwired: 2 in, 2 out]
                n199 = property on="Test Slider" class="Slide (strict)"("Visible"=FALSE) -> ()  [unwired: 2 in, 2 out]
              }
              frame "Exposure Priority  **" {
                n200 = Index Array(array=w336, index=3) -> (element=w337:cluster{string[]})
                n201 = call <vilib>:"NT Read String.vi"("Name"=w339) -> ("String"=w338:string)  [unwired: 9 in, 1 out]
                n202 = Unbundle(w337) -> (w333:string[])
                n203 = Match First String(2:w333, 3:w338) -> (0:w334:i32)  [unwired: 1 out]
                n204 = property on="Test Ring" class="Ring (strict)"("Value"=w334, "Strings []"=w333) -> ()  [unwired: 2 in, 2 out]
                n205 = property on="Test Ring" class="Ring (strict)"("Visible"=TRUE) -> ()  [unwired: 2 in, 2 out]
                n206 = property on="Test Slider" class="Slide (strict)"("Visible"=FALSE) -> ()  [unwired: 2 in, 2 out]
              }
              frame "Color Enable  **" {
                n207 = Index Array(array=w345, index=4) -> (element=w346:cluster{string[]})
                n208 = call <vilib>:"NT Read String.vi"("Name"=w348) -> ("String"=w347:string)  [unwired: 9 in, 1 out]
                n209 = Unbundle(w346) -> (w342:string[])
                n210 = Match First String(2:w342, 3:w347) -> (0:w343:i32)  [unwired: 1 out]
                n211 = property on="Test Ring" class="Ring (strict)"("Value"=w343, "Strings []"=w342) -> ()  [unwired: 2 in, 2 out]
                n212 = property on="Test Ring" class="Ring (strict)"("Visible"=TRUE) -> ()  [unwired: 2 in, 2 out]
                n213 = property on="Test Slider" class="Slide (strict)"("Visible"=FALSE) -> ()  [unwired: 2 in, 2 out]
              }
              frame Default {
                n214 = property on="Test Ring" class="Ring (strict)"("Visible"=FALSE) -> ()  [unwired: 2 in, 2 out]
                n215 = property on="Test Slider" class="Slide (strict)"("Visible"=FALSE) -> ()  [unwired: 2 in, 2 out]
              }
              frame "Brightness  **", "Color Level  **", "Compression  **", "FPS  **", "Sharpness  **" {
                n216 = call <vilib>:"NT Read Number.vi"("Name"=w354) -> ("Numeric"=w353:dbl)  [unwired: 9 in, 1 out]
                n217 = local write "Test Slider"(w353) -> ()
                n218 = property on="Test Slider" class="Slide (strict)"("Visible"=TRUE, "Scale.Maximum"=100.0 ("Scale.Range:Maximum")) -> ()  [unwired: 2 in, 2 out]
                n219 = property on="Test Ring" class="Ring (strict)"("Visible"=FALSE) -> ()  [unwired: 2 in, 2 out]
              }
            }
          }
        }
        n220 = property on="Progress" class="Clust (strict)"("Visible"=FALSE) -> ()  [unwired: 2 in, 2 out]
      }
      event "Test Name": Mouse Enter {
        # "Populate the ring with the list of tests"
        n221 = event-data() -> ()  [unwired: 1 in, 1 out]
        n222 = call <vilib>:"NT Read String Array.vi"("Name"="TestMode/TestList") -> ("String Array"=w362:string[])  [unwired: 9 in, 1 out]
        n223 = Build Array (concatenate)("Select the test to run...", w362) -> (w361:string[])
        n224 = property on="Test Name" class="Ring (strict)"("Strings []"=w361) -> ()  [unwired: 2 in, 2 out]
      }
      event "Test Name": Value Change {
        w364 = FALSE ("Visible")
        # "Tell the robot the test name to run"
        n225 = event-data() -> ("NewVal"=w368:u16)  [unwired: 1 in]
        n226 = property on="Test Name" class="Ring (strict)"() -> ("Strings []"=w369:string[])  [unwired: 2 in, 2 out]
        n227 = local write "Progress"(T8 {"Test Progress"=0, "Test Progress Text"=""} ("Progress")) -> ()
        n228 = Index Array(array=w369, index=w368) -> (element=w367:string)
        n229 = call <vilib>:"NT Write String.vi"("String"=w367, "Name"="TestMode/TestName") -> ()  [unwired: 9 in, 1 out]
        n230 = property on="Progress" class="Clust (strict)"("Visible"=TRUE) -> ()  [unwired: 2 in, 2 out]
        n231 = property on="Motor" class="Clust (strict)"("Visible"=w364) -> ()  [unwired: 2 in, 2 out]
        n232 = property on="Test Slider" class="Slide (strict)"("Visible"=w364) -> ()  [unwired: 2 in, 2 out]
        n233 = property on="On/Off" class="Bool (strict)"("Visible"=w364) -> ()  [unwired: 2 in, 2 out]
        n234 = property on="Rev/Fwd" class="Clust (strict)"("Visible"=w364) -> ()  [unwired: 2 in, 2 out]
        n235 = property on="Test Ring" class="Ring (strict)"("Visible"=w364) -> ()  [unwired: 2 in, 2 out]
      }
      event "Select Auto": Mouse Enter {
        # "Populate the combo box with the list of autonomous options"
        n236 = event-data() -> ()  [unwired: 1 in, 1 out]
        n237 = call <vilib>:"NT Read String Array.vi"("Name"="Auto List") -> ("String Array"=w371:string[])  [unwired: 9 in, 1 out]
        n238 = property on="Select Auto" class="CmbBox"("Strings[]"=w371) -> ()  [unwired: 2 in, 2 out]
      }
      event "Select Auto": Value Change {
        # "User modified the Auto Selection. Write to NT variable so robot knows."
        n239 = event-data() -> ("NewVal"=w374:string)  [unwired: 1 in]
        n240 = call <vilib>:"NT Write String.vi"("String"=w374, "Name"="Auto Selector") -> ()  [unwired: 9 in, 1 out]
      }
      event "Command Selection": Value Change {
        # "Get the params and show in table"
        n241 = event-data() -> ("NewVal"=w380:i32)  [unwired: 1 in]
        n242 = property on="Command Selection" class="MCListbox (strict)"() -> ("ItemNames"=w378:string[][])  [unwired: 2 in, 2 out]
        n243 = call <vilib>:"WPI_DashboardUpdate Command Params.vi"("NewVal"=w380, "Commands"=w378, "Param Tbl"=w379) -> ()  [unwired: 8 in, 1 out]
      }
      event "Execute Command": Value Change {
        # "Started one, Unique ID holds\nresponse"
        n244 = event-data() -> ()  [unwired: 1 in, 1 out]
        n245 = property on="Command Selection" class="MCListbox (strict)"() -> ("ItemNames"=w391:string[][])  [unwired: 2 in, 2 out]
        n246 = Index Array(array=w391, index (row)="Command Selection", index (col)=0) -> (element=w389:string)
        n247 = call <vilib>:"Invoke Commands.vi"("Command Params"="Command Params", "Function Name"=w389) -> ("Params"=w385:u8, "Started"=w384:bool)  [unwired: 7 in, 1 out]
        n248 = Array Subset(array="Command Params", length (row)=w385) -> (w386:string[][])  [unwired: 3 in]
        n249 = Select(t="Executing" ("Cmd Status"), s=w384, f="" ("Cmd Status")) -> (s? t:f=→"Cmd Status":string)
      }
      event "Command Selection": Double Click {
        n250 = event-data() -> ("Row"=w399:i32)  [unwired: 1 in]
        n251 = property on="Command Selection" class="MCListbox (strict)"() -> ("ItemNames"=w402:string[][])  [unwired: 2 in, 2 out]
        n252 = local read "Command Params"() -> (w398:string[][])
        n253 = Index Array(array=w402, index (row)=w399, index (col)=0) -> (element=w400:string)
        n254 = call <vilib>:"Invoke Commands.vi"("Command Params"=w398, "Function Name"=w400) -> ("Params"=w397:u8, "Started"=w392:bool)  [unwired: 7 in, 1 out]
        n255 = Array Subset(array=w398, length (row)=w397) -> (w396:string[][])  [unwired: 3 in]
        n256 = Select(t="Executing" ("Cmd Status"), s=w392, f="" ("Cmd Status")) -> (s? t:f=w393:string)
        n257 = local write "Cmd Status"(w393) -> ()
      }
      event "CheckList": Double Click {
        # "Shift clears all"
        # "Update symbols on the listbox"
        n258 = event-data() -> ("PlatMods.Shift"=w404:bool, "Row"=w406:i32)  [unwired: 1 in]
        n259 = case shown="True" w404 {
          tunnel: w406 -> [w410 _]
          tunnel: 1 -> [w409 _]
          frame False {
            n260 = property on="CheckList" class="LstBox (strict)"() -> ("Item Symbols"=w408:i32[])  [unwired: 2 in, 2 out]
            n261 = Replace Array Subset(array=w408, new element=w409, index=w410) -> (w407:i32[])
            n262 = property on="CheckList" class="LstBox (strict)"("Item Symbols"=w407) -> ()  [unwired: 2 in, 2 out]
          }
          frame True {
            w411 = 0 ("Top Row")
            n263 = property on="CheckList" class="LstBox (strict)"() -> ("Number of Rows"=w413:u32)  [unwired: 2 in, 2 out]
            n264 = Initialize Array(0, w413) -> (w412:i32[])
            n265 = property on="CheckList" class="LstBox (strict)"("Top Row"=w411, "Value"=w411, "Item Symbols"=w412) -> ()  [unwired: 2 in, 2 out]
          }
        }
      }
      event "CheckList": Key Down {
        # "Update symbols on the listbox\nLeft and right keys check and uncheck"
        n266 = event-data() -> ("VKey"=w417:T24)  [unwired: 1 in]
        n267 = case shown="\"Left\", \"Right\"" w417 {
          selector: w417 -> [w422 _]
          tunnel: eventvkey."Left" ("VKey") -> [w420 _]
          frame "Left", "Right" {
            n268 = Equal?(x=w420, y=w422) -> (x = y?=w421:bool)
            n269 = Select(t=0, s=w421, f=1) -> (s? t:f=w423:i32)
            n270 = property on="CheckList" class="LstBox (strict)"() -> ("Item Symbols"=w426:i32[])  [unwired: 2 in, 2 out]
            n271 = Replace Array Subset(array=w426, new element=w423, index="CheckList") -> (w425:i32[])
            n272 = property on="CheckList" class="LstBox (strict)"("Item Symbols"=w425) -> ()  [unwired: 2 in, 2 out]
          }
          frame Default {
          }
        }
      }
      event "Motor.Enable": Value Change {
        # "When the test mode otor enable helper is set, update that\ntree row item's value"
        n273 = event-data() -> ("NewVal"=w432:bool)  [unwired: 1 in]
        n274 = Unbundle("Motor") -> ("Value"=w431:dbl)  [unwired: 1 out]
        n275 = Select(t=w431, s=w432, f=0.0) -> (s? t:f=w429:dbl)
        n276 = call <vilib>:"NT Write Number.vi"("Numeric"=w429, "Name"=w428) -> ()  [unwired: 9 in, 1 out]
      }
      event "Test Slider": Value Change {
        # "When the test mode slider helper is set, update that\ntree row item's value"
        n277 = event-data() -> ("NewVal"=w435:dbl)  [unwired: 1 in]
        n278 = call <vilib>:"NT Write Number.vi"("Numeric"=w435, "Name"=w436) -> ()  [unwired: 9 in, 1 out]
      }
      event "On/Off": Value Change {
        # "When the test mode on/off helper value is set, update that\ntree row item's value"
        n279 = event-data() -> ("NewVal"=w440:bool)  [unwired: 1 in]
        n280 = Boolean To (0,1)(Boolean=w440) -> (0, 1=w439:i16)
        n281 = call <vilib>:"NT Write Number.vi"("Numeric"=w439, "Name"=w438) -> ()  [unwired: 9 in, 1 out]
      }
      event "Rev/Fwd": Value Change {
        # "When the test mode helper value for relays is set, update that\ntree row item's value"
        n282 = event-data() -> ("NewVal.Forward"=w448:bool, "NewVal.Reverse"=w447:bool)  [unwired: 1 in]
        n283 = Boolean To (0,1)(Boolean=w448) -> (0, 1=w444:i16)
        n284 = Boolean To (0,1)(Boolean=w447) -> (0, 1=w446:i16)
        n285 = Negate(x=w446) -> (-x=w445:i16)
        n286 = Add(x=w444, y=w445) -> (x+y=w443:i16)
        n287 = call <vilib>:"NT Write Number.vi"("Numeric"=w443, "Name"=w442) -> ()  [unwired: 9 in, 1 out]
      }
      event "Test Ring": Value Change {
        # "When a test mode helper value is selected from the ring,\nset the tree item's variable to the string value"
        n288 = event-data() -> ("NewVal"=w452:u16)  [unwired: 1 in]
        n289 = property on="Test Ring" class="Ring (strict)"() -> ("Strings []"=w453:string[])  [unwired: 2 in, 2 out]
        n290 = Index Array(array=w453, index=w452) -> (element=w451:string)
        n291 = call <vilib>:"NT Write String.vi"("String"=w451, "Name"=w450) -> ()  [unwired: 9 in, 1 out]
      }
      event "Rec Mode": Value Change {
        # "Update globals for recording mode and path to read log from.\nClear when logging and let NetworkTables set path for vision to\nuse."
        n292 = event-data() -> ("NewVal"=w464:enum32{"Stop", "Record", "Playback"})  [unwired: 1 in]
        n293 = global write "WPI_DashboardLogging Global.vi" "Logging Filename"(path "") -> ()
        n294 = global write "WPI_DashboardLogging Global.vi" "Recording"(w464) -> ()
        n295 = case shown="\"Playback\"" w464 {
          tunnel: w463 -> [_ w466 w475]
          tunnel: [_ _ w474] -> w461
          tunnel: [_ _ w473] -> _
          tunnel: w459 -> [_ _ w471]
          tunnel: cluster{i32, i32} {-250, 170} -> [_ _ w470]
          tunnel: [_ _ T25 {"Image Size"=TRUE, "Image Type"=TRUE, "Pixel Value"=TRUE, "ROI Information"=TRUE, "Zoom Factor"=FALSE} ("Image Information Shown:All Elements")] -> w454
          tunnel: [_ _ TRUE ("Zoom Factor")] -> w455
          tunnel: w457 -> [_ _ w467]
          frame Default {
          }
          frame "Stop", "Record" {
            # "Place Window too"
            n296 = invoke class="VI" method="FP.Close"(reference=w466) -> (reference out=w465:refnum<vi>)  [unwired: 2 in, 2 out]
            n297 = invoke class="VI" method="Abort VI"(reference=w465) -> ()  [unwired: 2 in, 3 out]
          }
          frame "Playback" {
            n298 = call "Open Playback Panel.vi"("Offset"=w470, "DB VI Ref"=w471, "Playback in"=w475) -> ("Playback out"=w472:refnum<vi>)  [unwired: 8 in]
            n299 = register-events(w472, w467) -> (reference out=w474:refnum<event-registration>, error out=w473:errorcluster)  [unwired: 2 in]
          }
        }
        n300 = property on="Camera Image Right" class="ImageControl"("Image Information Shown"=w454, "Image Information Visible"=w455) -> ()  [unwired: 2 in, 2 out]
        n301 = property on="Camera Image" class="ImageControl"("Image Information Shown"=w454, "Image Information Visible"=w455) -> ()  [unwired: 2 in, 2 out]
        n302 = call <vilib>:"WPI_DashboardNT Log FieldName Cache.vi"("Operation"=enum16{"Lookup/Add", "Index", "Clear"}."Clear") -> ()  [unwired: 8 in, 3 out]
      }
      event Panel Close {
        w477 = enum32{"Stop", "Record", "Playback"}."Stop" ("Rec Mode")
        # "Playback window has been closed, abort"
        n303 = event-data() -> ()  [unwired: 1 in, 4 out]
        n304 = local write "Rec Mode"(w477) -> ()
        n305 = global write "WPI_DashboardLogging Global.vi" "Recording"(w477) -> ()
      }
      event Panel Close {
        # "Abort playback window and ourself"
        n306 = event-data() -> ()  [unwired: 1 in, 4 out]
        n307 = invoke class="VI" method="FP.Close"(reference=w481) -> (reference out=w480:refnum<vi>)  [unwired: 2 in, 2 out]
        n308 = invoke class="VI" method="Abort VI"(reference=w480) -> (error out=w479:errorcluster)  [unwired: 2 in, 2 out]
        n309 = invoke class="VI" method="Abort VI"(error in=w479) -> ()  [unwired: 2 in, 3 out]
      }
      event User Event {
        n310 = event-data() -> ("IDs"=w488:cluster{"RPC field ID":u16, "Unique ID":u16}, "String"=w487:string)  [unwired: 1 in]
        n311 = Bundle("IDs"=w488, "String"=w487) -> (w486:T11)  [unwired: 1 in]
        n312 = call <vilib>:"Retrieve RPC Response.vi"("RPC Response"=w486) -> ("Output"=w484:string[][])  [unwired: 10 in]
        n313 = Build Array (concatenate)(w482, w484) -> (w483:string[][])
        n314 = local write "Command Params"(w483) -> ()
        n315 = local write "Cmd Status"("" ("Cmd Status")) -> ()
      }
      event "Tree": Double Click {
        n316 = event-data() -> ("PlatMods"=w494:T28, "Tag"=w491:string)  [unwired: 1 in]
        n317 = Unbundle(w494) -> ("Shift"=w493:bool)  [unwired: 4 out]
        n318 = String Subset(string=w491, length (rest)=1 ("length (rest)")) -> (substring=w490:string)  [unwired: 1 in]
        n319 = Not(x=w493) -> (.not. x?=w492:bool)
        n320 = case shown="\"/\"" w490 {
          tunnel: w491 -> [_ w497]
          tunnel: w492 -> [_ w496]
          frame Default {
          }
          frame "/" {
            n321 = call <vilib>:"NT Update Persistence.vi"("Persistence"=w496, "Name"=w497) -> ()  [unwired: 9 in, 1 out]
          }
        }
      }
    }
  }
  n322 = while {
    tunnel: w65 -> [w499]
    i -> [w502]
    stop <- FALSE stop-if-true
    n323 = Wait (ms)(milliseconds to wait=u32 100) -> ()  [unwired: 1 out]
    n324 = case shown="\"Playback\"" "Rec Mode" {
      tunnel: w502 -> [_ _ w517]
      tunnel: [u32 2829099 ("Base Color") u32 11141120 ("Target Color") w506] -> w498
      frame "Stop", Default {
        # "Reset the color, extra updates don't cost much"
      }
      frame "Record" {
      }
      frame "Playback" {
        # "Playback"
        n325 = Quotient & Remainder(x=w517, y=u32 50 ("milliseconds to wait")) -> (x-y*floor(x/y)=w513:u32)  [unwired: 1 out]
        n326 = Divide(x=w513, y=u32 50 ("milliseconds to wait")) -> (x/y=w510:dbl)
        n327 = Multiply(x=6.283185307179586, y=w510) -> (x*y=w515:dbl)
        n328 = Sine(x=w515) -> (sin(x)=w514:dbl)
        n329 = Absolute Value(x=w514) -> (abs(x)=w507:dbl)
        n330 = call "Interpolate RGB Color.vi"("Proportion"=w507, "Target Color"=u32 30976, "Base Color"=u32 2829099) -> ("Result Color"=w506:u32)  [unwired: 8 in]
      }
    }
    n331 = property class="Pane"(reference=w499, "PaneColor"=w498) -> ()  [unwired: 1 in, 2 out]
  }
  n332 = local write "Dashboard Tab"(T2."Drive" ("Dashboard Tab")) -> ()
  n333 = property on="On/Off" class="Bool (strict)"("Visible"=w36) -> ()  [unwired: 2 in, 2 out]
  n334 = property on="Motor" class="Clust (strict)"("Visible"=w36) -> ()  [unwired: 2 in, 2 out]
  n335 = property on="Progress" class="Clust (strict)"("Visible"=w36) -> ()  [unwired: 2 in, 2 out]
  n336 = property on="Test Ring" class="Ring (strict)"("Visible"=w36) -> ()  [unwired: 2 in, 2 out]
  n337 = property on="Rev/Fwd" class="Clust (strict)"("Visible"=w36) -> ()  [unwired: 2 in, 2 out]
  n338 = while {
    tunnel: u16 1741 ("timeout ms (25000)") -> [w519]
    stop <- FALSE stop-if-true
    n339 = TCP Create Listener(10:w519) -> (0:w518:errorcluster, 3:w520:refnum<k5>)  [unwired: 4 in, 1 out]
    n340 = case shown="No Error" w518 {
      selector: w518 -> [w522 _]
      tunnel: w520 -> [w523 _]
      frame No Error {
        n341 = while {
          tunnel: w523 -> [w526]
          tunnel: w522 -> [w525]
          stop <- FALSE stop-if-true
          n342 = TCP Wait On Listener(8:w525, 11:w526) -> (0:w527:errorcluster, 4:w528:refnum<k5>)  [unwired: 2 in, 3 out]
          n343 = local write "TCP"(w528) -> ()
          n344 = case shown="No Error" w527 {
            frame No Error {
            }
            frame Error {
              n345 = Wait (ms)(milliseconds to wait=u32 1000) -> ()  [unwired: 1 out]
            }
          }
        }
      }
      frame Error {
        n346 = Wait (ms)(milliseconds to wait=u32 1000) -> ()  [unwired: 1 out]
      }
    }
  }
  n347 = local write "Command Selection"(u16 0 ("milliseconds to wait")) -> ()
  n348 = local write "Command Params"(string[][] [] ("Command Params")) -> ()
  n349 = global write "WPI_DashboardLogging Global.vi" "Recording"(w59) -> ()
  n350 = local write "Rec Mode"(w59) -> ()
  n351 = call <vilib>:"NT Write String.vi"("String"="Select Auto", "Name"="Auto Selector") -> ()  [unwired: 9 in, 1 out]
